vi "Current slew rate.vi"() -> ()   [LabVIEW 2021]
doc: "Current slew rate.vi helps user to control current slew rate of the Programmable Power Supply."
uses:
  <instrlib>/niDCPower/nidcpower.llb/niDCPower Wait For Event - Event.ctl
  <instrlib>/niDCPower/nidcpower.llb/niDCPower Source Mode.ctl
  <instrlib>/niDCPower/nidcpower.llb/niDCPower Output Function.ctl
  <instrlib>/niDCPower/nidcpower.llb/niDCPower Aperture Time Units.ctl
  <instrlib>/niScope/Controls/niScope trigger slope.ctl
  <instrlib>/niScope/Utility/niScope Get Channel Name From String.vi
  <instrlib>/niScope/Configure/Trigger/niScope Configure Trigger Digital.vi
  <instrlib>/niDCPower/nidcpower.llb/niDCPower Configure Digital Edge Measure Trigger With Channels.vi
  <instrlib>/niScope/Acquire/Fetch/niScope Fetch WDT.vi
panel:
  in  "MeasGraphs":T1(tab)
  out "CurrentV/STime":waveform(dbl)(graph) caption="Load Transient"
  in  "SourceOutput Voltage v/s Time":string="SOURCE CURRENT vs TIME"
  out "Error status":string
  out "ScopeAmplitudeV/STime":waveform(dbl)(graph) caption="Load Transient"
  in  "ScopeOutput Voltage v/s Time":string="SCOPE AMPLITUDE vs TIME"
  in  "Error in":errorcluster caption="error in (no error)"
  out "Error out":errorcluster caption="error out"
  in  "MeasConfigurations":enum32{"Source Config", "Scope Config"}(tab)
  in  "TransientResponseTab":T2(tab)
  in  "Source transient response":i32(ring)=1038 caption="TRANSIENT RESPONSE" items=["Slow"=1041, "Normal"=1038, "Fast"=1039, "Custom"=1042]
  in  "Source current gain bandwidth":dbl=40000.0 caption="GAIN BANDWIDTH" format="%#_6pHz"
  in  "Source current compensation frequency":dbl=4000.0 caption="COMP. FREQUENCY" format="%#_6pHz"
  in  "Source current pole-zero ratio":dbl=1.0 caption="POLE-ZERO RATIO"
  in  "Source update rate":dbl=1000.0 caption="UPDATE RATE" format="%#_6pS/s"
  in  "Source sense":i32(ring)=1009 caption="SENSE" items=["Local"=1008, "Remote"=1009]
  in  "Source current C2 time":dbl=0.005 caption="TIME for C2" format="%#_6ps"
  in  "Source current C1 time":dbl=0.005 caption="TIME for C1" format="%#_6ps"
  in  "Source current slew rate":dbl=500.0 caption="CURRENT SLEW RATE" format="%#_6pA/s"
  in  "Source voltage limit range":dbl=20.0 caption="VOLTAGE LIMIT RANGE" format="%#_6pV"
  in  "Source current level range":dbl=3.0 caption="CURRENT LEVEL RANGE" format="%#_6pA"
  in  "Source current set point 2(C2)":dbl=3.0 caption="CURRENT SET POINT 2" format="%#_6pA"
  in  "Source current set point 1(C1)":dbl caption="CURRENT SET POINT 1" format="%#_6pA"
  in  "Source resource name":refnum<k15> caption="RESOURCE NAME"
  in  "Source SourceAdapt":string="Current SourceAdapt Parameters"
  in  "Source sample rate":dbl=1800000.0 caption="SAMPLE RATE" format="%#_6pS/s"
  out "Expected time for source to achevie slew rate":dbl caption="EXPECTED TIME FOR SLEW RATE" format="%#_6ps"
  in  "Scope enable/disable":bool caption="Scope Enable/Disable"
  in  "Scope vertical range":dbl=10.0 caption="VERTICAL RANGE"
  in  "Scope resourceName":refnum<k15> caption="RESOURCE NAME"
  in  "Scope probe attenuation":dbl=1.0 caption="PROBE ATTENUATION"
  in  "Scope sample rate":dbl=1800000.0 caption="SAMPLE RATE" format="%#_6pHz"
  in  "Scope output channel name":string="0" caption="INPUT CHANNEL NAME"
  in  "Scope vertical coupling":enum32{"AC", "DC"}(ring)=enum."DC" caption="VERTICAL COUPLING"
  # "CURRENT SLEW RATE"
  # "-"
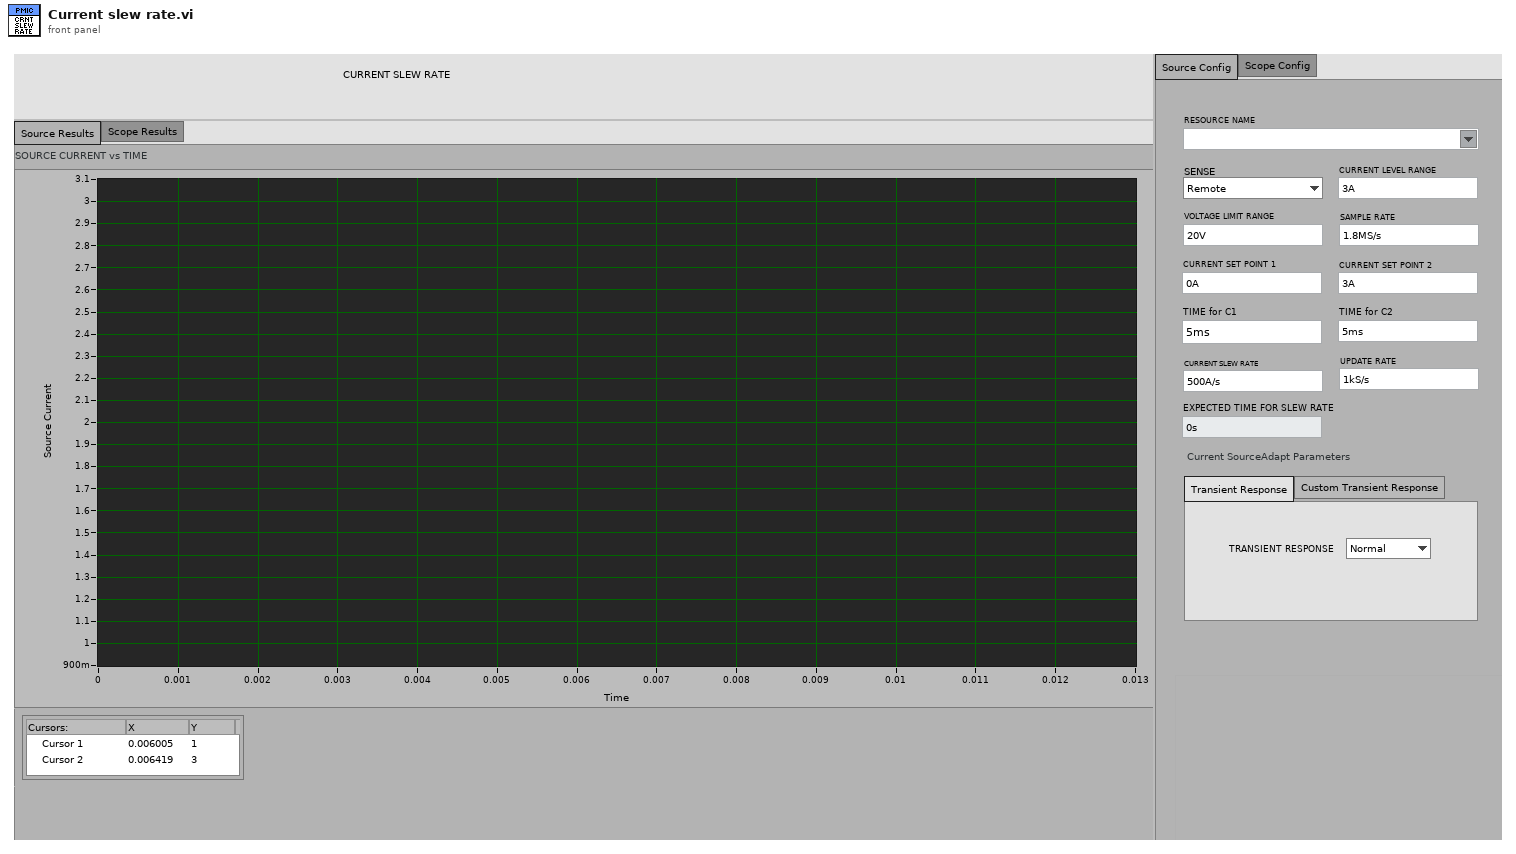
[diagram p1: front panel]
types:
  T1 = enum32{"Source Results", "Scope Results", "Hidden Controls"}
  T2 = enum32{"Transient Response", "Custom Transient Response"}
  T3 = typedef "niDCPower Aperture Time Units.ctl" = i32
  T4 = typedef "niDCPower Output Function.ctl" = i32
  T5 = typedef "niDCPower Wait For Event - Event.ctl" = i32
  T6 = typedef "niDCPower Source Mode.ctl" = i32
  T7 = typedef "niScope trigger slope.ctl" = i32
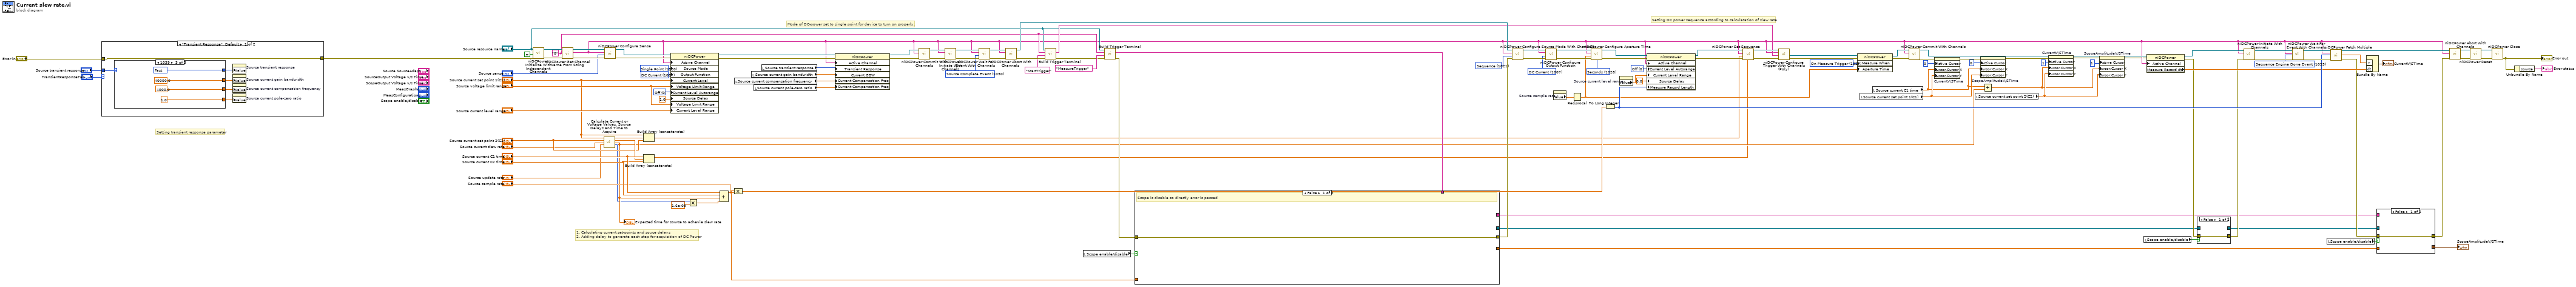
[diagram p0: block diagram]
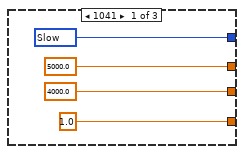
[diagram p2: hidden frame]
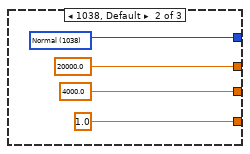
[diagram p3: hidden frame]
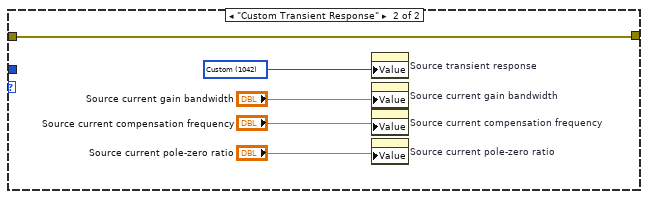
[diagram p4: hidden frame]
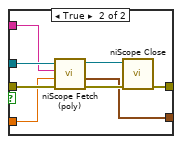
[diagram p5: hidden frame]
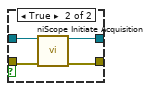
[diagram p6: hidden frame]
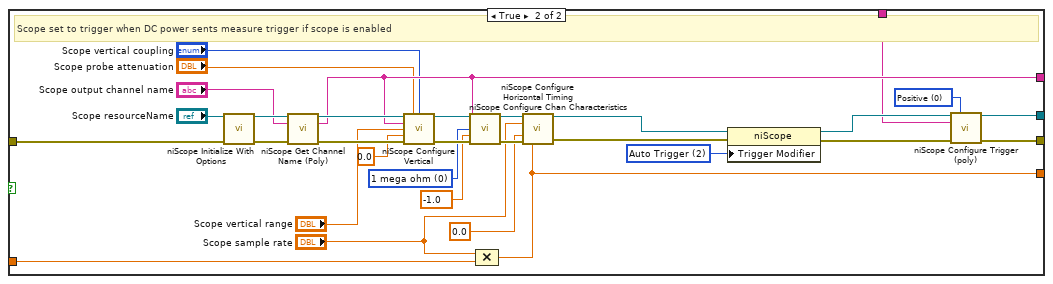
[diagram p7: hidden frame]
diagram:
  w87 = 1027 items=["Automatically after Source Complete"=1025, "On Demand"=1026, "On Measure Trigger"=1027] ("Measurement:Advanced:Measure When")
  w90 = 0 items=["Off", "On"] ("Source:DC Current:Current Level Autorange")
  w95 = T3 1028 items=["Seconds"=1028, "Powerline Cycles"=1029] ("aperture time units")
  w94 = T4 1007 items=["DC Voltage"=1006, "DC Current"=1007, "Pulse Voltage"=1049, "Pulse Current"=1050] ("output function")
  w96 = T5 1033 items=["Source Complete Event"=1030, "Measure Complete Event"=1031, "Sequence Iteration Complete Event"=1032, "Sequence Engine Done Event"=1033, "Pulse Complete Event"=1051, "Ready For Pulse Trigger Event"=1052] ("event")
  w97 = T6 1021 items=["Single Point"=1020, "Sequence"=1021] ("source mode")
  w61 = "0" ("index")
  w115 = 0 items=["Off", "On"] ("Source:DC Current:Current Level Autorange")
  w124 = T5 1030 items=["Source Complete Event"=1030, "Measure Complete Event"=1031, "Sequence Iteration Complete Event"=1032, "Sequence Engine Done Event"=1033, "Pulse Complete Event"=1051, "Ready For Pulse Trigger Event"=1052] ("event")
  w127 = 1007 items=["DC Voltage"=1006, "DC Current"=1007, "Pulse Voltage"=1049, "Pulse Current"=1050] ("Source:Output Function")
  w128 = 1020 items=["Single Point"=1020, "Sequence"=1021] ("Source:Source Mode")
  # "1. Calculating current set-points and souce delays\n2. Adding delay to generate each step for acquisition of DC Power"
  # "Setting DC power sequence according to calculatation of slew rate"
  # "Mode of DC-power set to single point for device to turn on properly."
  # "Setting transient response parameter"
  n1 = case shown="\"Transient Response\", Default" "TransientResponseTab" {
    tunnel: "Error in" -> [w130 w147]
    tunnel: [w130 w147] -> w31
    tunnel: "Source transient response" -> [w129 _]
    frame "Transient Response", Default {
      n2 = case shown="1039" w129 {
        tunnel: [w138 w142 w146] -> w134
        tunnel: [5000.0 ("Source voltage gain bandwidth") 20000.0 ("Source voltage gain bandwidth") 40000.0 ("Source voltage gain bandwidth")] -> w133
        tunnel: [4000.0 ("Source voltage compensation frequency") 4000.0 ("Source voltage compensation frequency") 4000.0 ("Source voltage compensation frequency")] -> w131
        tunnel: [1.0 ("Source voltage pole-zero ratio") 1.0 ("Source voltage pole-zero ratio") 1.0 ("Source voltage pole-zero ratio")] -> w132
        frame 1041 {
          w138 = 1041 items=["Slow"=1041, "Normal"=1038, "Fast"=1039, "Custom"=1042] ("Source transient response")
        }
        frame 1038, Default {
          w142 = 1038 items=["Slow"=1041, "Normal"=1038, "Fast"=1039, "Custom"=1042] ("Source transient response")
        }
        frame 1039 {
          w146 = 1039 items=["Slow"=1041, "Normal"=1038, "Fast"=1039, "Custom"=1042] ("Source transient response")
        }
      }
      n3 = property on="Source transient response" class="Ring (strict)"("Value"=w134) -> ()  [unwired: 2 in, 2 out]
      n4 = property on="Source current gain bandwidth" class="DigNum (strict)"("Value"=w133) -> ()  [unwired: 2 in, 2 out]
      n5 = property on="Source current compensation frequency" class="DigNum (strict)"("Value"=w131) -> ()  [unwired: 2 in, 2 out]
      n6 = property on="Source current pole-zero ratio" class="DigNum (strict)"("Value"=w132) -> ()  [unwired: 2 in, 2 out]
    }
    frame "Custom Transient Response" {
      w151 = 1042 items=["Slow"=1041, "Normal"=1038, "Fast"=1039, "Custom"=1042] ("Source transient response")
      n7 = property on="Source transient response" class="Ring (strict)"("Value"=w151) -> ()  [unwired: 2 in, 2 out]
      n8 = property on="Source current gain bandwidth" class="DigNum (strict)"("Value"="Source current gain bandwidth") -> ()  [unwired: 2 in, 2 out]
      n9 = property on="Source current compensation frequency" class="DigNum (strict)"("Value"="Source current compensation frequency") -> ()  [unwired: 2 in, 2 out]
      n10 = property on="Source current pole-zero ratio" class="DigNum (strict)"("Value"="Source current pole-zero ratio") -> ()  [unwired: 2 in, 2 out]
    }
  }
  n11 = call <instrlib>:"niDCPower Initialize With Independent Channels.vi"("error in (no error)"=w31, "reset (false)"=TRUE, "resource name"="Source resource name") -> ("error out"=w109:errorcluster, "instrument handle out"=w112:refnum<k15>)  [unwired: 7 in]
  n12 = call <instrlib>:"niDCPower Get Channel Name From String.vi"("error in (no error)"=w109, "index"=w61, "instrument handle"=w112) -> ("error out"=w110:errorcluster, "name"=w25:string, "instrument handle out"=w111:refnum<k15>)  [unwired: 6 in]
  n13 = call "Calculate Current or Voltage Values, Source Delays and Time to Acquire.vi"("Current/voltage start point (AorV)"="Source current set point 1(C1)", "Current/voltage end point (AorV)"="Source current set point 2(C2)", "Current/voltage slew rate (AorV/sec)"="Source current slew rate", "Update Rate (S/sec)"="Source update rate") -> ("Current or voltage values"=w8:dbl[], "Source delays (sec)"=w7:dbl[], "Time to acquire (sec)"=w3:dbl, "Number of samples"=w2:i32)  [unwired: 7 in, 1 out]
  "Expected time for source to achevie slew rate" <- w3
  n14 = call <instrlib>:"niDCPower Configure Sense.vi"("error in (no error)"=w110, "sense"="Source sense", "channel name"=w25, "instrument handle"=w111) -> ("error out"=w120:errorcluster, "instrument handle out"=w121:refnum<k15>)  [unwired: 6 in]
  n15 = Build Array (concatenate)("Source current set point 1(C1)", w8, "Source current set point 2(C2)") -> (w26:dbl[])
  n16 = Build Array (concatenate)("Source current C1 time", w7, "Source current C2 time") -> (w1:dbl[])
  n17 = property class="niDCPower"(reference=w121, error in=w120, "Active Channel"=w25, "Source Mode"=w128, "Output Function"=w127, "Current Level"="Source current set point 1(C1)", "Voltage Limit Range"="Source voltage limit range", "Current Level Autorange"=w115, "Source Delay"=1.0 ("Source:Advanced:Source Delay"), "Voltage Limit Range"="Source voltage limit range", "Current Level Range"="Source current level range") -> (reference out=w117:refnum<k15>, error out=w116:errorcluster)
  n18 = Multiply(x=w2, y=1.6e-05) -> (x*y=w23:dbl)
  n19 = Compound Arithmetic op=ADD("Source current C1 time", "Source current C2 time", w3, w23) -> (w64:dbl)
  n20 = local read "Source current compensation frequency"() -> (w39:dbl)
  n21 = Compound Arithmetic op=MULTIPLY("Source sample rate", w64) -> (w104:dbl)
  n22 = local read "Source current gain bandwidth"() -> (w40:dbl)
  n23 = local read "Source current pole-zero ratio"() -> (w38:dbl)
  n24 = local read "Source transient response"() -> (w37:i32)
  n25 = property class="niDCPower"(reference=w117, error in=w116, "Active Channel"=w25, "Transient Response"=w37, "Current GBW"=w40, "Current Compensation Freq"=w39, "Current Compensation Freq"=w38) -> (reference out=w114:refnum<k15>, error out=w113:errorcluster)
  n26 = call <instrlib>:"niDCPower Commit With Channels.vi"("error in (no error)"=w113, "channel name"=w25, "instrument handle"=w114) -> ("error out"=w118:errorcluster, "instrument handle out"=w119:refnum<k15>)  [unwired: 7 in]
  n27 = call <instrlib>:"niDCPower Initiate With Channels.vi"("error in (no error)"=w118, "channel name"=w25, "instrument handle"=w119) -> ("error out"=w126:errorcluster, "instrument handle out"=w125:refnum<k15>)  [unwired: 7 in]
  n28 = call <instrlib>:"niDCPower Wait For Event With Channels.vi"("error in (no error)"=w126, "event"=w124, "channel name"=w25, "instrument handle"=w125) -> ("error out"=w123:errorcluster, "instrument handle out"=w122:refnum<k15>)  [unwired: 6 in]
  n29 = call <instrlib>:"niDCPower Abort With Channels.vi"("error in (no error)"=w123, "channel name"=w25, "instrument handle"=w122) -> ("error out"=w75:errorcluster, "instrument handle out"=w82:refnum<k15>)  [unwired: 7 in]
  n30 = call "Build Trigger Terminal.vi"("error in (no error)"=w75, "Trigger/Event Name"="StartTrigger" ("Trigger Type"), "Channel Name"=w61, "Resource Name"="Source resource name") -> ("error out"=w51:errorcluster, "Terminal Name"=w74:string)  [unwired: 6 in]
  n31 = local read "Scope enable/disable"() -> (w41:bool)
  n32 = call "Build Trigger Terminal.vi"("error in (no error)"=w51, "Trigger/Event Name"="MeasureTrigger", "Channel Name"=w61, "Resource Name"="Source resource name") -> ("error out"=w62:errorcluster, "Terminal Name"=w54:string)  [unwired: 6 in]
  n33 = case shown="False" w41 {
    tunnel: [w152 w165] -> w72
    tunnel: [_ w164] -> w67
    tunnel: [_ w163] -> w65
    tunnel: w64 -> [_ w162]
    tunnel: [_ w161] -> w63
    tunnel: w62 -> [w152 w160]
    tunnel: w54 -> [_ w159]
    frame False {
      # "Scope is disable so directly error is passed"
    }
    frame True {
      w172 = 2 items=["None"=1, "Auto Trigger"=2] ("Trigger Modifier")
      w168 = u32 0 items=["1 mega ohm"=0, "50 ohms"=2] ("Input Impedance")
      w169 = T7 0 items=["Positive", "Negative"] ("trigger slope")
      # "Scope set to trigger when DC power sents measure trigger if scope is enabled"
      n34 = call <instrlib>:"niScope Initialize With Options.vi"("resource name"="Scope resourceName", "error in"=w160) -> ("instrument handle"=w183:refnum<k15>, "error out"=w182:errorcluster)  [unwired: 12 in]
      n35 = call-poly <instrlib>:"niScope Get Channel Name (Poly).vi"("instrument handle"=w183, "index"="Scope output channel name", "error in"=w182) -> ("instrument handle out"=w171:refnum<k15>, "channel name"=w163:string, "error out"=w170:errorcluster)  [unwired: 10 in]
      n36 = call <instrlib>:"niScope Configure Vertical.vi"("instrument handle"=w171, "probe attenuation"="Scope probe attenuation", "vertical coupling"="Scope vertical coupling", "channels"=w163, "vertical range"="Scope vertical range", "vertical offset"=0.0, "error in"=w170) -> ("instrument handle out"=w181:refnum<k15>, "error out"=w180:errorcluster)  [unwired: 7 in]
      n37 = call <instrlib>:"niScope Configure Chan Characteristics.vi"("instrument handle"=w181, "channels"=w163, "input impedance"=w168, "maximum input frequency"=-1.0 ("Maximum Input Frequency"), "error in"=w180) -> ("instrument handle out"=w178:refnum<k15>, "error out"=w179:errorcluster)  [unwired: 9 in]
      n38 = Compound Arithmetic op=MULTIPLY("Scope sample rate", w162) -> (w161:dbl)
      n39 = call <instrlib>:"niScope Configure Horizontal Timing.vi"("instrument handle"=w178, "min sample rate"="Scope sample rate", "reference position"=0.0 ("Reference Position"), "error in"=w179, "min record length"=w161) -> ("instrument handle out"=w175:refnum<k15>, "error out"=w174:errorcluster)  [unwired: 9 in]
      n40 = property on="Property Node" class="niScope"(reference=w175, error in=w174, "Trigger Modifier"=w172) -> (reference out=w166:refnum<k15>, error out=w173:errorcluster)
      n41 = call-poly <instrlib>:"niScope Configure Trigger (poly).vi"("instrument handle"=w166, "trigger slope"=w169, "trigger source"=w159, "error in"=w173) -> ("instrument handle out"=w164:refnum<k15>, "error out"=w165:errorcluster)  [unwired: 10 in]
    }
  }
  n42 = call <instrlib>:"niDCPower Configure Source Mode With Channels.vi"("error in (no error)"=w72, "source mode"=w97, "channel name"=w25, "instrument handle"=w82) -> ("error out"=w100:errorcluster, "instrument handle out"=w99:refnum<k15>)  [unwired: 6 in]
  n43 = call <instrlib>:"niDCPower Configure Output Function.vi"("error in (no error)"=w100, "output function"=w94, "channel name"=w25, "instrument handle"=w99) -> ("error out"=w102:errorcluster, "instrument handle out"=w101:refnum<k15>)  [unwired: 6 in]
  n44 = property on="Source sample rate" class="DigNum (strict)"() -> ("Value"=w34:dbl)  [unwired: 2 in, 2 out]
  n45 = Reciprocal(x=w34) -> (1/x=w53:dbl)
  n46 = call <instrlib>:"niDCPower Configure Aperture Time.vi"("aperture time units"=w95, "error in (no error)"=w102, "aperture time"=w53, "channel name"=w25, "instrument handle"=w101) -> ("error out"=w92:errorcluster, "instrument handle out"=w91:refnum<k15>)  [unwired: 5 in]
  n47 = To Long Integer(number=w104) -> (32bit integer=w79:i32)
  n48 = property on="Source current level range" class="DigNum (strict)"() -> ("Value"=w35:dbl)  [unwired: 2 in, 2 out]
  n49 = property class="niDCPower"(reference=w91, error in=w92, "Active Channel"=w25, "Current Level Autorange"=w90, "Current Level Range"=w35, "Source Delay"=0.0 ("Source:Advanced:Source Delay"), "Measure Record Length"=w79) -> (reference out=w107:refnum<k15>, error out=w108:errorcluster)
  n50 = call <instrlib>:"niDCPower Set Sequence.vi"("source delays"=w1, "error in (no error)"=w108, "values"=w26, "channel name"=w25, "instrument handle"=w107) -> ("error out"=w88:errorcluster, "instrument handle out"=w89:refnum<k15>)  [unwired: 5 in]
  n51 = call-poly <instrlib>:"niDCPower Configure Trigger With Channels (Poly).vi"("error in (no error)"=w88, "input terminal"=w74, "channel name"=w25, "instrument handle"=w89) -> ("error out"=w84:errorcluster, "instrument handle out"=w86:refnum<k15>)  [unwired: 6 in]
  n52 = property class="niDCPower"(reference=w86, error in=w84, "Measure When"=w87, "Aperture Time"=w53) -> (reference out=w85:refnum<k15>, error out=w83:errorcluster)
  n53 = local read "Source current set point 1(C1)"() -> (w17:dbl)
  n54 = local read "Source current C1 time"() -> (w10:dbl)
  n55 = call <instrlib>:"niDCPower Commit With Channels.vi"("error in (no error)"=w83, "channel name"=w25, "instrument handle"=w85) -> ("error out"=w22:errorcluster, "instrument handle out"=w103:refnum<k15>)  [unwired: 7 in]
  n56 = property on="CurrentV/STime" class="WFGraph (strict)"(error in=w22, "Active Cursor"=u32 0, "Cursor.Cursor X"=w10, "Cursor.Cursor Y"=w17) -> (error out=w21:errorcluster)  [unwired: 1 in, 1 out]
  n57 = local read "Source current set point 2(C2)"() -> (w16:dbl)
  n58 = property on="ScopeAmplitudeV/STime" class="WFGraph (strict)"(error in=w21, "Active Cursor"=u32 0, "Cursor.Cursor X"=w10, "Cursor.Cursor Y"=w17) -> (error out=w20:errorcluster)  [unwired: 1 in, 1 out]
  n59 = Add(x=w10, y=w3) -> (x+y=w11:dbl)
  n60 = property on="CurrentV/STime" class="WFGraph (strict)"(error in=w20, "Active Cursor"=u32 1, "Cursor.Cursor X"=w11, "Cursor.Cursor Y"=w16) -> (error out=w19:errorcluster)  [unwired: 1 in, 1 out]
  n61 = property on="ScopeAmplitudeV/STime" class="WFGraph (strict)"(error in=w19, "Active Cursor"=u32 1, "Cursor.Cursor X"=w11, "Cursor.Cursor Y"=w16) -> (error out=w18:errorcluster)  [unwired: 1 in, 1 out]
  n62 = local read "Scope enable/disable"() -> (w43:bool)
  n63 = property class="niDCPower"(reference=w103, error in=w18, "Active Channel"=w25) -> (reference out=w98:refnum<k15>, error out=w71:errorcluster, "Measure Record dt"=w77:dbl)
  n64 = case shown="False" w43 {
    tunnel: w71 -> [w184 w188]
    tunnel: [w184 w187] -> w70
    tunnel: w67 -> [_ w186]
    tunnel: [_ w185] -> w66
    frame False {
    }
    frame True {
      n65 = call <instrlib>:"niScope Initiate Acquisition.vi"("instrument handle"=w186, "error in"=w188) -> ("instrument handle out"=w185:refnum<k15>, "error out"=w187:errorcluster)  [unwired: 12 in]
    }
  }
  n66 = call <instrlib>:"niDCPower Initiate With Channels.vi"("error in (no error)"=w70, "channel name"=w25, "instrument handle"=w98) -> ("error out"=w106:errorcluster, "instrument handle out"=w105:refnum<k15>)  [unwired: 7 in]
  n67 = call <instrlib>:"niDCPower Wait For Event With Channels.vi"("error in (no error)"=w106, "event"=w96, "channel name"=w25, "instrument handle"=w105) -> ("error out"=w81:errorcluster, "instrument handle out"=w80:refnum<k15>)  [unwired: 6 in]
  n68 = local read "Scope enable/disable"() -> (w42:bool)
  n69 = call <instrlib>:"niDCPower Fetch Multiple.vi"("instrument handle"=w80, "channel name"=w25, "count (1)"=w79, "error in (no error)"=w81) -> ("instrument handle out"=w78:refnum<k15>, "current measurements"=w76:dbl[], "error out"=w69:errorcluster)  [unwired: 6 in, 3 out]
  n70 = Bundle By Name("Y"=w76, "dt"=w77) -> (→"CurrentV/STime":waveform(dbl))  [unwired: 1 in]
  n71 = case shown="False" w42 {
    tunnel: w69 -> [w189 w197]
    tunnel: [w189 w196] -> w68
    tunnel: w66 -> [_ w194]
    tunnel: w65 -> [_ w193]
    tunnel: w63 -> [_ w191]
    tunnel: [_ w190] -> w27
    frame False {
    }
    frame True {
      n72 = call-poly <instrlib>:"niScope Fetch (poly).vi"("error in"=w197, "numSamples"=w191, "channels"=w193, "instrument handle"=w194) -> ("error out"=w195:errorcluster, "wfm"=w190:waveform(dbl), "instrument handle out"=w192:refnum<k15>)  [unwired: 4 in, 1 out]
      n73 = call <instrlib>:"niScope Close.vi"("instrument handle"=w192, "error in"=w195) -> ("error out"=w196:errorcluster)  [unwired: 13 in]
    }
  }
  "ScopeAmplitudeV/STime" <- w27
  n74 = call <instrlib>:"niDCPower Abort With Channels.vi"("error in (no error)"=w68, "channel name"=w25, "instrument handle"=w78) -> ("error out"=w59:errorcluster, "instrument handle out"=w57:refnum<k15>)  [unwired: 7 in]
  n75 = call <instrlib>:"niDCPower Reset.vi"("error in (no error)"=w59, "instrument handle"=w57) -> ("error out"=w58:errorcluster, "instrument handle out"=w56:refnum<k15>)  [unwired: 8 in]
  n76 = call <instrlib>:"niDCPower Close.vi"("error in (no error)"=w58, "instrument handle"=w56) -> ("error out"=w29:errorcluster)  [unwired: 9 out]
  "Error out" <- w29
  n77 = Unbundle By Name(w29) -> ("source"=→"Error status":string)
